vi "using_DAC_sub_vi.vi"() -> ()   [LabVIEW 2012]
panel:
  in  "manager":T1={"address"="localhost", "port"=7682, "password"=""}
  in  "update":bool
  in  "Channel":cluster{string, dbl}={"comp1", 1.0}
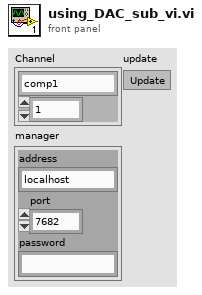
[diagram p1: front panel]
types:
  T1 = cluster{"address":string, "port":u16, "password":string}
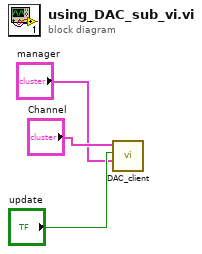
[diagram p0: block diagram]
diagram:
  n1 = call "DAC_client.vi"("manager"="manager", "update"="update", "Channel"="Channel") -> ()  [unwired: 9 in]
